vi "unwrapFFT.vi"(4 "phase offset":dbl format="%#_13g", 7 "active col":i32, 8 "sequence NBXZ":dbl[][](array[numeric])=[[0.0, 4.0], [0.0, 4.0], [0.0, 4.0], [0.0, 4.0]], 9 "phase array":dbl[](array[numeric])=[0.0, 0.25, 0.5, 0.75], 10 "fft cluster":T1, 11 "result array IN":dbl[][](array[numeric])) -> (0 "Intensity Graph":dbl[][](graph), 1 "FFT array":dbl[][](array[numeric]))   [LabVIEW 2018, in "myFFT.lvlib"]
uses:
  <vilib>/Analysis/2dsp.llb/2D Inverse Complex FFT.vi
  myFFT.lvlib
  <vilib>/Analysis/NI_AALPro.lvlib
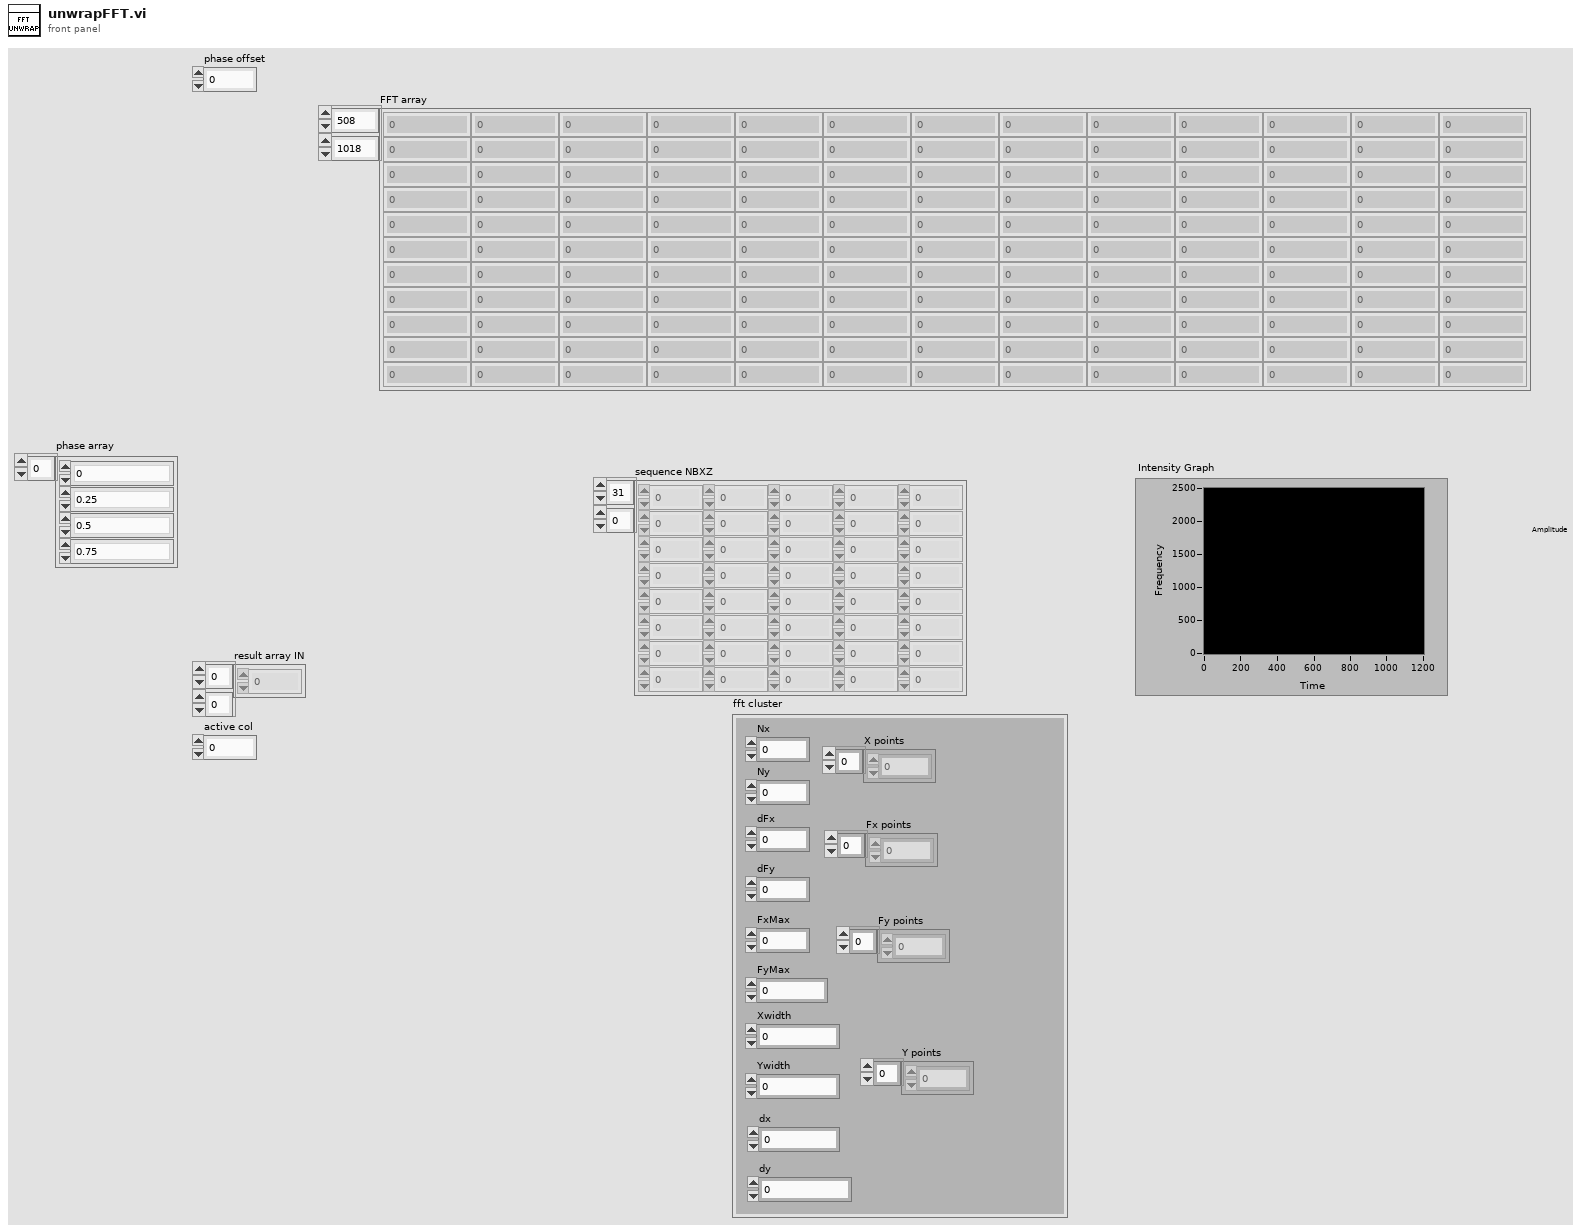
[diagram p1: front panel]
types:
  T1 = cluster{"dFx":dbl, "dFy":dbl, "Nx":i32, "Ny":i32, "FxMax":dbl, "FyMax":dbl, "Xwidth":dbl, "Ywidth":dbl, "dx":dbl, "dy":dbl, "Fx points":dbl[], "X points":dbl[], "Y points":dbl[], "Fy points":dbl[]}
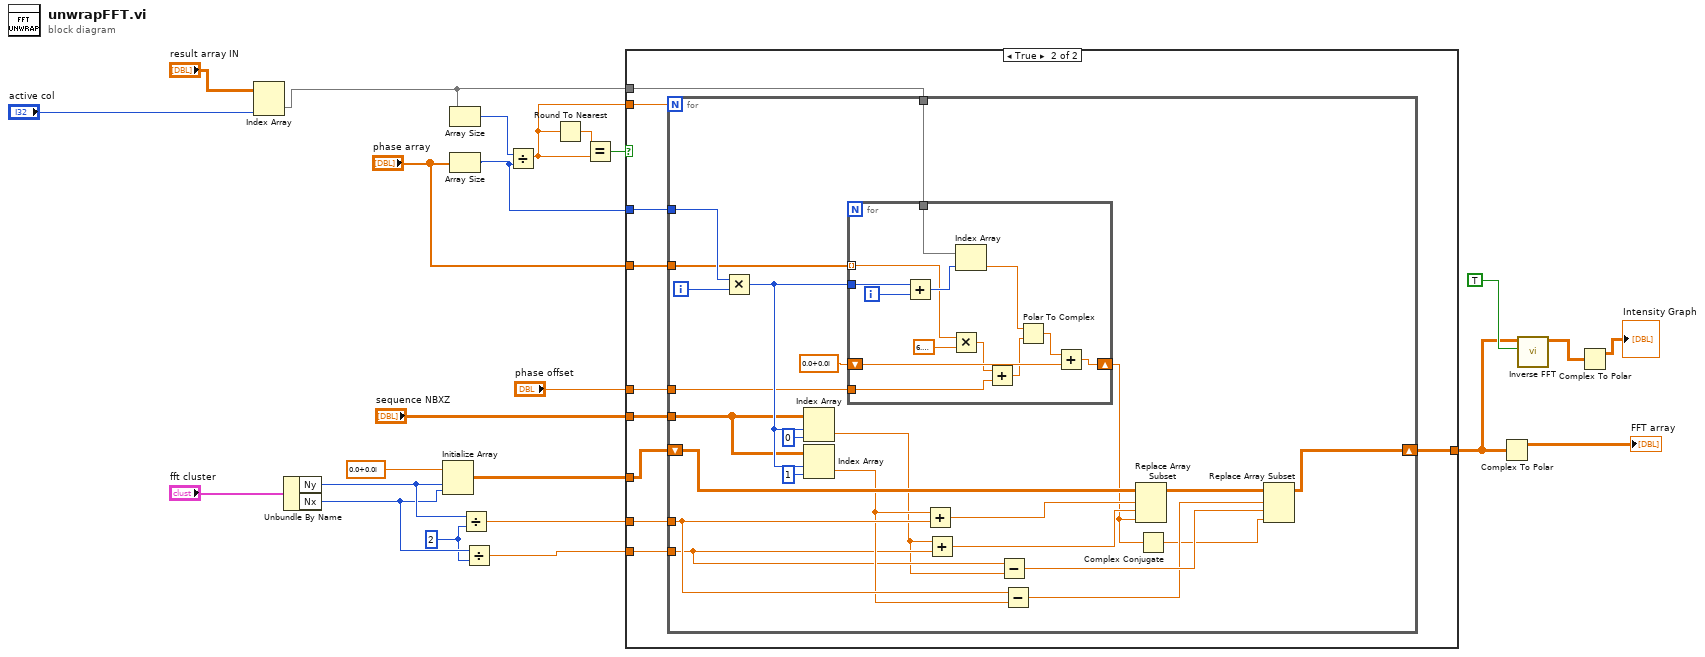
[diagram p0: block diagram]
diagram:
  w13 = 2 ("y")
  n1 = Index Array(array="result array IN", index (col)="active col") -> (element=w2:dbl[])  [unwired: 1 in]
  n2 = Unbundle By Name("fft cluster") -> ("Ny"=w15:i32, "Nx"=w14:i32)
  n3 = Initialize Array(cdb 0.0+0.0i, w15, w14) -> (w16:cdb[][])
  n4 = Array Size(array=w2) -> (size(s)=w24:i32)
  n5 = Array Size(array="phase array") -> (size(s)=w20:i32)
  n6 = Divide(x=w15, y=w13) -> (x/y=w12:dbl)
  n7 = Divide(x=w14, y=w13) -> (x/y=w11:dbl)
  n8 = Divide(x=w24, y=w20) -> (x/y=w21:dbl)
  n9 = Round To Nearest(number=w21) -> (nearest integer value=w23:dbl)
  n10 = Equal?(x=w23, y=w21) -> (x = y?=w22:bool)
  n11 = case shown="True" w22 {
    tunnel: w21 -> [_ w34]
    tunnel: w20 -> [_ w33]
    tunnel: w2 -> [_ w32]
    tunnel: "phase array" -> [_ w31]
    tunnel: "sequence NBXZ" -> [_ w30]
    tunnel: w16 -> [_ w29]
    tunnel: [_ w28] -> w7
    tunnel: w12 -> [_ w27]
    tunnel: w11 -> [_ w26]
    tunnel: "phase offset" -> [_ w25]
    frame False {
    }
    frame True {
      n12 = for {
        N: w34 -> [_]
        tunnel: w33 -> [w56]
        tunnel: w32 -> [w55]
        tunnel: w31 -> [w54]
        tunnel: w30 -> [w49]
        shift-right: [w44] -> w28
        shift-left: w29 -> [w48]
        tunnel: w27 -> [w43]
        tunnel: w26 -> [w41]
        tunnel: w25 -> [w35]
        i -> [w57]
        n13 = Multiply(x=w56, y=w57) -> (x*y=w51:i32)
        n14 = Index Array(array=w49, index (row)=w51, index (col)=0 ("disabled index (col)")) -> (element=w40:dbl)
        n15 = Index Array(array=w49, index (row)=w51, index (col)=1 ("disabled index (col)")) -> (element=w42:dbl)
        n16 = for {
          tunnel: w51 -> [w69]
          tunnel: w55 -> [w68]
          tunnel: w54 -> [w61] mode=indexing
          shift-right: [w63] -> w37
          shift-left: cdb 0.0+0.0i -> [w62]
          tunnel: w35 -> [w58]
          i -> [w70]
          n17 = Add(x=w69, y=w70) -> (x+y=w67:i32)
          n18 = Multiply(x=w61, y=6.283185307179586) -> (x*y=w60:dbl)
          n19 = Index Array(array=w68, index=w67) -> (element=w65:dbl)
          n20 = Add(x=w60, y=w58) -> (x+y=w59:dbl)
          n21 = Polar To Complex(1:w59, 2:w65) -> (0:w64:cdb)
          n22 = Add(x=w64, y=w62) -> (x+y=w63:cdb)
        }
        n23 = Add(x=w42, y=w43) -> (x+y=w47:dbl)
        n24 = Add(x=w40, y=w41) -> (x+y=w46:dbl)
        n25 = Subtract(x=w41, y=w40) -> (x-y=w39:dbl)
        n26 = Subtract(x=w43, y=w42) -> (x-y=w38:dbl)
        n27 = Replace Array Subset(array=w48, new element=w37, index (row)=w47, index (col)=w46) -> (w45:cdb[][])
        n28 = Complex Conjugate(1:w37) -> (0:w36:cdb)
        n29 = Replace Array Subset(array=w45, new element=w36, index (row)=w38, index (col)=w39) -> (w44:cdb[][])
      }
    }
  }
  n30 = Complex To Polar(r * e^(i*theta)=w7) -> (r=→"FFT array":dbl[][])  [unwired: 1 out]
  n31 = call-poly <vilib>:"Inverse FFT.vi"("shift?"=TRUE, "FFT {x}"=w7) -> ("X"=w10:cdb[][])  [unwired: 8 in, 1 out]
  n32 = Complex To Polar(r * e^(i*theta)=w10) -> (r=→"Intensity Graph":dbl[][])  [unwired: 1 out]
